vi "test_ni_lm_optimization.vi"() -> ()   [LabVIEW 2019]
panel:
  out "XY Graph":cluster{"Angles":dbl[], "Intensities":dbl[]}[](graph)
  out "best fit parameters":dbl[](array[numeric])
  out "best nonlinear fit":dbl[](array[numeric])
  in  "Intensities":dbl[](array[numeric])
  in  "Angles":dbl[](array[numeric])
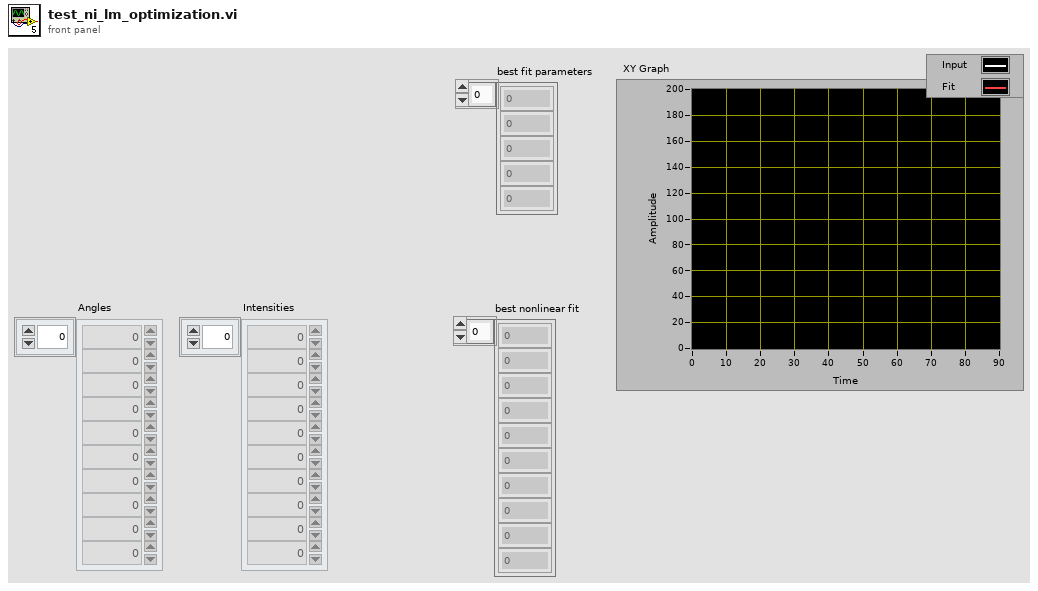
[diagram p1: front panel]
types:
  T1 = cluster{"Angles":dbl[], "best nonlinear fit":dbl[]}
  T2 = cluster{"Angles":dbl[], "best nonlinear fit":dbl[]}[]
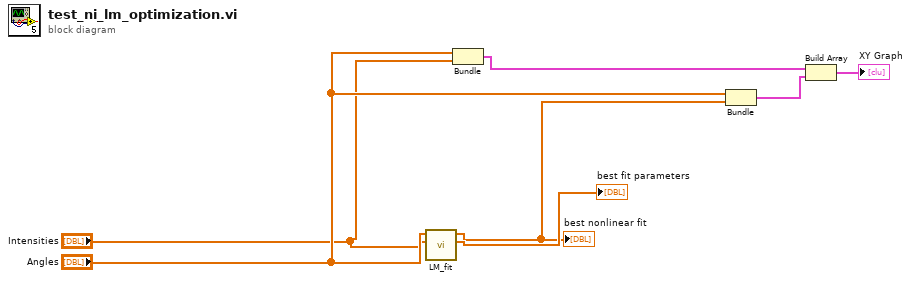
[diagram p0: block diagram]
diagram:
  n1 = call "LM_fit.vi"("Intensities"="Intensities", "Angles"="Angles") -> ("best fit parameters"=→"best fit parameters":dbl[], "best nonlinear fit"=w2:dbl[])  [unwired: 7 in, 1 out]
  "best nonlinear fit" <- w2
  n2 = Bundle("Angles"="Angles", "Intensities"="Intensities") -> (w6:cluster{"Angles":dbl[], "Intensities":dbl[]})  [unwired: 1 in]
  n3 = Bundle("Angles"="Angles", "best nonlinear fit"=w2) -> (w1:T1)  [unwired: 1 in]
  n4 = Build Array(w6, w1) -> (→"XY Graph":T2)
